vi "SCPI Read Upper Limits.vi"(8 "error in (no error)":errorcluster, 11 "VISA resource name":refnum<visa-resource-name>) -> (0 "error out":errorcluster, 1 "Set Current":dbl format="%.2g", 2 "Set Voltage":dbl format="%.2g", 3 "VISA resource name out":refnum<visa-resource-name>)   [LabVIEW 2021, in "BK Precision 169XB.lvlib"]
doc: "Returns the actual voltage level and actual current level for a desired channel."
uses:
  BK Precision 169XB.lvlib
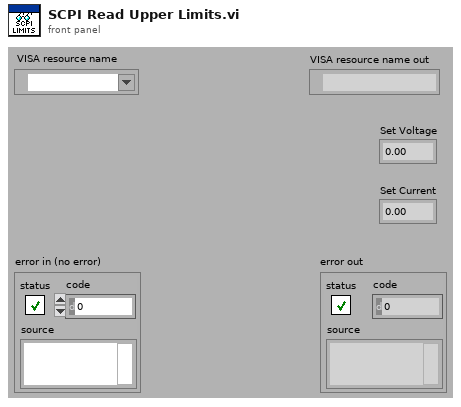
[diagram p1: front panel]
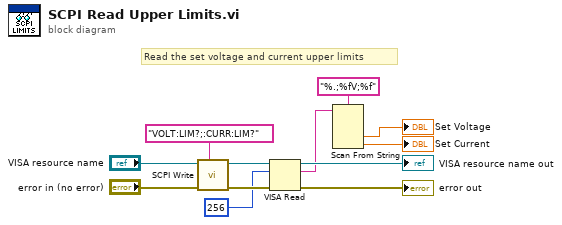
[diagram p0: block diagram]
diagram:
  # "Read the set voltage and current upper limits"
  n1 = call "SCPI Write.vi"("Input String"="VOLT:LIM?;:CURR:LIM?", "error in (no error)"="error in (no error)", "VISA resource name"="VISA resource name") -> ("error out"=w10:errorcluster, "VISA resource name out"=w9:refnum<visa-resource-name>)  [unwired: 7 in]
  n2 = VISA Read(VISA resource name=w9, byte count=u32 256, error in (no error)=w10) -> (VISA resource name out=→"VISA resource name out":refnum<visa-resource-name>, read buffer=w5:string, error out=→"error out":errorcluster)  [unwired: 1 out]
  n3 = Scan From String(format string="%.;%fV;%f", input string=w5) -> (output 1=→"Set Voltage":dbl, output 2=→"Set Current":dbl)  [unwired: 4 in, 3 out]
